vi "Dummy.vi"() -> ()   [LabVIEW 2025, in "_Msg Rescript.lvlib" / "_Msg Rescript.lvclass"]
uses:
  _Msg Rescript.lvclass
  _Msg Rescript.lvclass/_Msg Rescript.ctl
panel:
  in  "Yes Msg Output in":refnum<class>
  out "Yes Msg Output out":refnum<class>
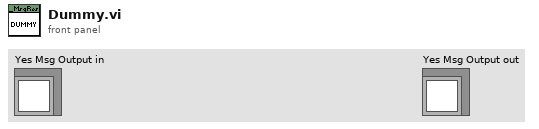
[diagram p1: front panel]
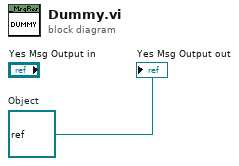
[diagram p0: block diagram]
diagram:
  w1 = refnum<class> refnum  # Object
  "Yes Msg Output out" <- w1
